vi "RESTful AttributeType To Text.vi"(1 "Service Attribute Type":T1=enum."Path") -> (0 "Boolean Text":string)   [LabVIEW 2020]
uses:
  <vilib>/AppBuilder/AB_Classes/RESTful/AB_RESTful_ServiceAttributeType.ctl
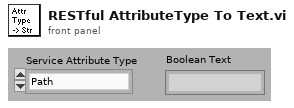
[diagram p1: front panel]
types:
  T1 = typedef "AB_RESTful_ServiceAttributeType.ctl" = enum32{"String", "Path"}
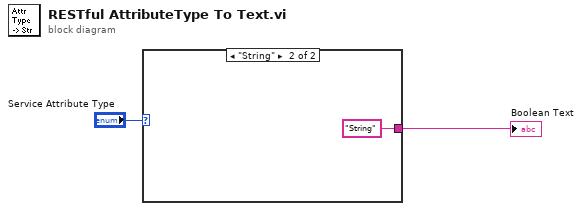
[diagram p0: block diagram]
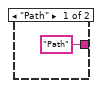
[diagram p2: hidden frame]
diagram:
  n1 = case shown="\"String\"" "Service Attribute Type" {
    tunnel: ["Path" ("Boolean Text") "String" ("Boolean Text")] -> w2
    frame "Path" {
    }
    frame "String" {
    }
  }
  "Boolean Text" <- w2
